vi "AllPartInfo_RC.vi"(8 "error in (no error)":errorcluster, 10 "AllPartInfo":T1=[{"PartName"="", "NumberOfRacks"=0, "MeasurementIDsArray"=[], "MeasurementNamesArray"=[], "SpecValuesArray"=[]}], 11 "Rack Controller in":refnum<class "Rack Controller.lvclass">) -> (0 "error out":errorcluster, 3 "Rack Controller out":refnum<class "Rack Controller.lvclass">)   [LabVIEW 2019, in "Rack Controller.lvclass"]
uses:
  Rack Controller.lvclass
  Common/Controls/AllPartInfo.ctl
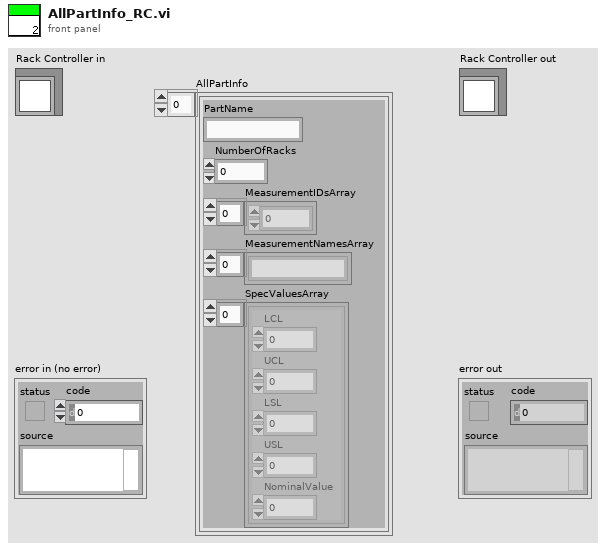
[diagram p1: front panel]
types:
  T1 = typedef "AllPartInfo.ctl" = cluster{"PartName":string, "NumberOfRacks":u8, "MeasurementIDsArray":u16[], "MeasurementNamesArray":string[], "SpecValuesArray":cluster{"LCL":dbl, "UCL":dbl, "LSL":dbl, "USL":dbl, "NominalValue":dbl}[]}[]
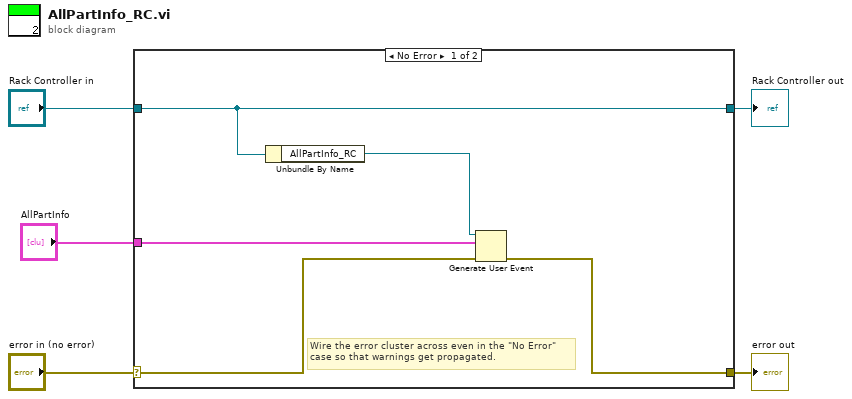
[diagram p0: block diagram]
diagram:
  n1 = case shown="No Error" "error in (no error)" {
    selector: "error in (no error)" -> [w9 w12]
    tunnel: [w8 w12] -> w4
    tunnel: [w10 w11] -> w2
    tunnel: "Rack Controller in" -> [w10 w11]
    tunnel: "AllPartInfo" -> [w6 _]
    frame No Error {
      # "Wire the error cluster across even in the \"No Error\"\ncase so that warnings get propagated."
      n2 = Unbundle By Name(w10) -> ("AllPartInfo_RC"=w7:refnum<user-event>)
      n3 = Generate User Event(user event=w7, event data cluster=w6, error in=w9) -> (error out=w8:errorcluster)  [unwired: 1 in, 1 out]
    }
    frame Error {
    }
  }
  "error out" <- w4
  "Rack Controller out" <- w2
